vi "Check Marker.vi"(7 "Maze":refnum<class "Maze.lvclass">, 8 "error in (no error)":errorcluster, 11 "Mouse in":refnum<class "Mouse.lvclass">) -> (0 "error out":errorcluster, 3 "Mouse out":refnum<class "Mouse.lvclass">)   [LabVIEW 2020, in "Maze.lvlib" / "Mouse.lvclass"]
uses:
  Mouse.lvclass
  Maze/Maze.lvclass
  Mouse.lvclass/Mouse.ctl
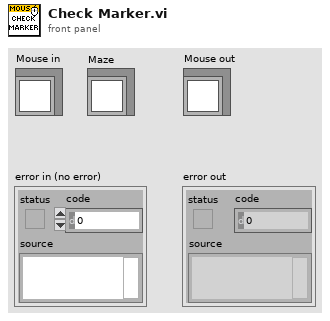
[diagram p1: front panel]
types:
  T1 = typedef "Maze.lvlib/Position.ctl" = cluster{"S":i32, "E":i32}
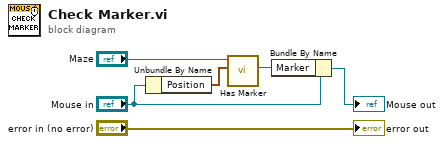
[diagram p0: block diagram]
diagram:
  n1 = Unbundle By Name("Mouse in") -> ("Position"=w4:T1)
  n2 = call "Has Marker.vi"("Position"=w4, "Maze in"="Maze") -> ("Has Marker?"=w2:bool)  [unwired: 7 in, 2 out]
  n3 = Bundle By Name(cluster="Mouse in", "Marker"=w2) -> (→"Mouse out":refnum<class "Mouse.lvclass">)
  "error out" <- "error in (no error)"
